vi "Device Name To ID.vi"(8 "Error In":errorcluster, 9 "Data":string, 10 "Device Name":string, 11 "Nest Config":T1) -> (0 "Error Out":errorcluster, 1 "Data":string, 2 "Device ID":string, 3 "Nest Config":T1)   [LabVIEW 2013, in "LMH-Nest.lvlib"]
doc: "Convert device name to device ID."
uses:
  LMH-Nest.lvlib
  Type Defs/Nest Config.ctl
  <vilib>/httpClient/ClientHandle.ctl
  Type Defs/Session Data.ctl
  Type Defs/Nest Error.ctl
  <vilib>/httpClient/LabVIEWHTTPClient.lvlib
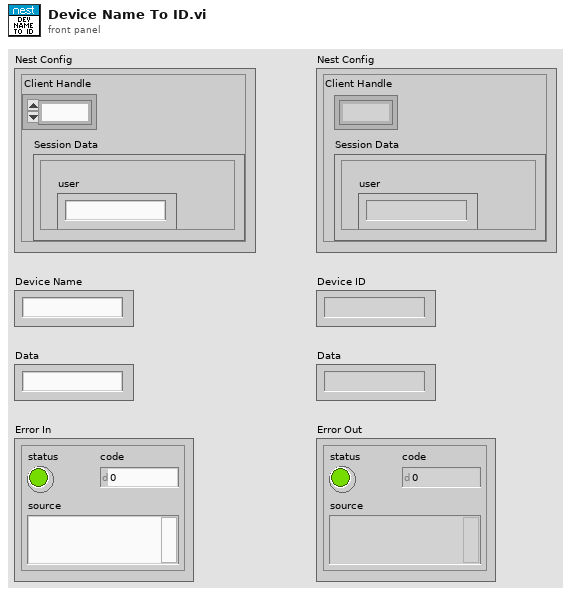
[diagram p1: front panel]
types:
  T1 = typedef "LMH-Nest.lvlib/Nest Config.ctl" = cluster{"Client Handle":T2, "Session Data":T3}
  T2 = typedef "LabVIEWHTTPClient.lvlib/ClientHandle.ctl" = refnum<k1>
  T3 = typedef "LMH-Nest.lvlib/Session Data.ctl" = cluster{"is_superuser":bool, "is_staff":bool, "urls":cluster{"transport_url":string, "rubyapi_url":string, "weather_url":string, "log_upload_url":string, "support_url":string}, "limits":cluster{"thermostats_per_structure":u32, "structures":u32, "thermostats":u32, "smoke_detectors":u32, "smoke_detectors_per_structure":u32}, "access_token":string, "userid":string, "expires_in":string, "email":string, "user":string, "language":string}
  T4 = typedef "LMH-Nest.lvlib/Nest Error.ctl" = enum16{"Unknown", "Auth", "Read", "Invalid Structure Name", "Invalid Device Name", "Set Temp"}
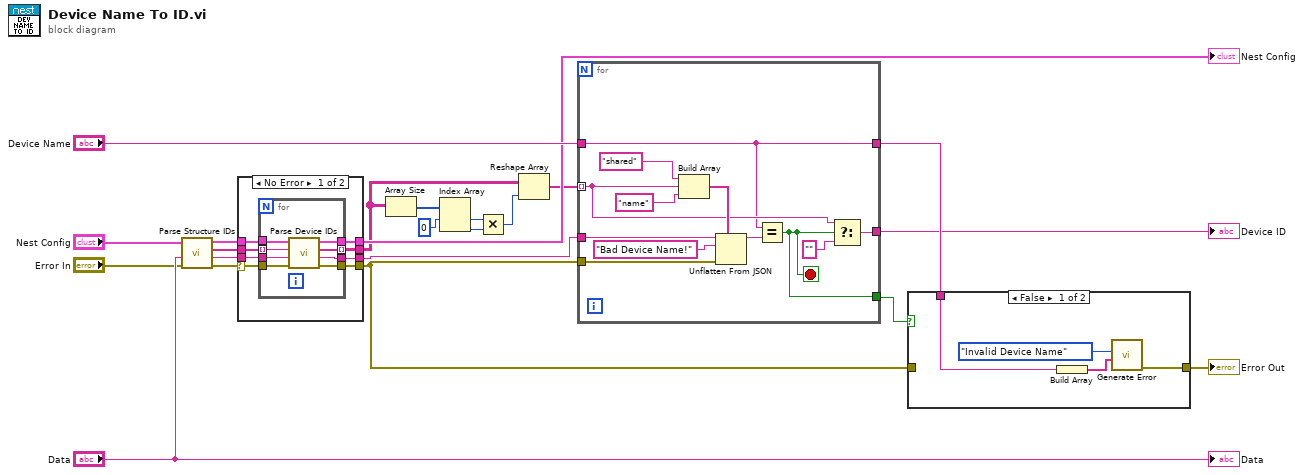
[diagram p0: block diagram]
diagram:
  n1 = call "Parse Structure IDs.vi"("Error In"="Error In", "Data"="Data", "Nest Config"="Nest Config") -> ("Error Out"=w11:errorcluster, "Data"=w17:string, "Structure IDs"=w16:string[], "Nest Config"=w15:T1)  [unwired: 5 in]
  n2 = case shown="No Error" w11 {
    selector: w11 -> [w23 w41]
    tunnel: w17 -> [w30 w39]
    tunnel: w16 -> [w29 _]
    tunnel: w15 -> [w28 w40]
    tunnel: [w27 w40] -> w14
    tunnel: [w26 _] -> w9
    tunnel: [w25 w39] -> w13
    tunnel: [w24 w41] -> w12
    frame No Error {
      n3 = for {
        tunnel: w23 -> [w38]
        tunnel: w30 -> [w37]
        tunnel: w29 -> [w36] mode=indexing
        tunnel: w28 -> [w35]
        tunnel: [w34] -> w27
        tunnel: [w33] -> w26 mode=indexing
        tunnel: [w32] -> w25
        tunnel: [w31] -> w24
        n4 = call "Parse Device IDs.vi"("Error In"=w38, "Data"=w37, "Structure ID"=w36, "Nest Config"=w35) -> ("Error Out"=w31:errorcluster, "Data"=w32:string, "Device IDs"=w33:string[], "Nest Config"=w34:T1)  [unwired: 4 in]
      }
    }
    frame Error {
    }
  }
  "Nest Config" <- w14
  n5 = Array Size(array=w9) -> (size(s)=w8:i32[])
  n6 = Index Array(array=w8, index #1=0 ("index")) -> (element #1=w6:i32, element #2=w5:i32)  [unwired: 1 in]
  n7 = Multiply(x=w6, y=w5) -> (x*y=w4:i32)
  n8 = Reshape Array(w9, w4) -> (w10:string[])
  n9 = for {
    tunnel: w12 -> [w50]
    tunnel: w10 -> [w46] mode=indexing
    tunnel: w13 -> [w49]
    tunnel: "Device Name" -> [w42]
    tunnel: [w44] -> w21
    tunnel: [w43] -> w18
    tunnel: [w42] -> w20
    stop <- w44 stop-if-true
    n10 = Build Array("shared", w46, "name" ("element")) -> (w51:string[])
    n11 = Unflatten From JSON(path=w51, JSON string=w49, type and defaults="Bad Device Name!" ("element"), error in (no error)=w50) -> (value=w47:string)  [unwired: 3 in, 1 out]
    n12 = Equal?(x=w42, y=w47) -> (x = y?=w44:bool)
    n13 = Select(t=w46, s=w44, f="") -> (s? t:f=w43:string)
  }
  "Device ID" <- w18
  n14 = case shown="False" w21 {
    tunnel: [w56 w58] -> w19
    tunnel: w20 -> [w55 _]
    tunnel: w12 -> [_ w58]
    frame False {
      n15 = Build Array(w55) -> (w54:string[])
      n16 = call "Generate Error.vi"("Args"=w54, "Nest Error"=Nest_Error."Invalid Device Name") -> ("Error Out"=w56:errorcluster)  [unwired: 9 in]
    }
    frame True {
    }
  }
  "Error Out" <- w19
  "Data" <- "Data"
